vi "testItemIndexOne.vi"(8 "error in (no error)":errorcluster, 11 "TestCase in":refnum<class "ListImp_Populated.lvclass">) -> (0 "error out":errorcluster, 3 "TestCase out":refnum<class "ListImp_Populated.lvclass">)   [LabVIEW 2013, in "ListImp_Populated.lvclass"]
uses:
  ListImp_Populated.lvclass
  ListImp_Populated.lvclass/ListImp_Populated.ctl
  source/LapDog.Collections.Lists/ListImp/ListImp.lvclass
  <vilib>/addons/_JKI Toolkits/VI Tester/TestCase.llb/TestCase.lvclass
  UnitTestComparisons/UnitTestComparisons.lvlib
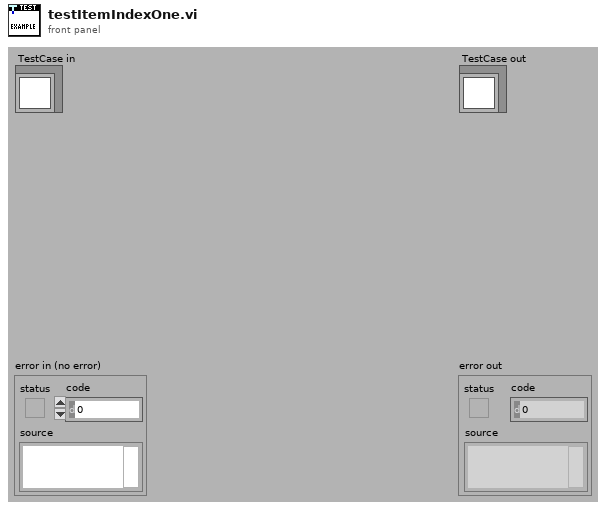
[diagram p1: front panel]
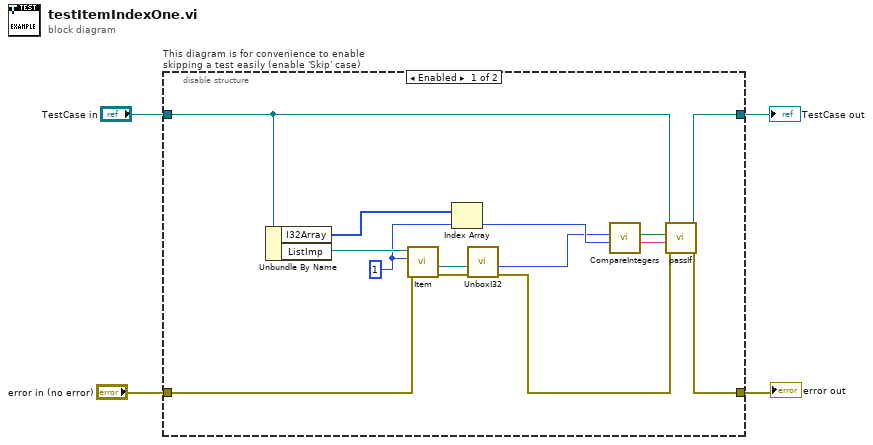
[diagram p0: block diagram]
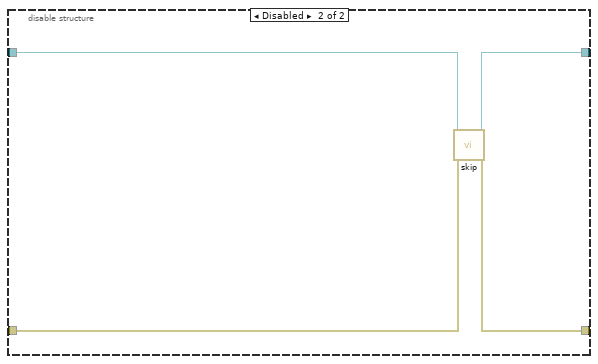
[diagram p2: hidden frame]
diagram:
  n1 = disable-structure "This diagram is for convenience to enable skipping a test easily (enable 'Skip' case)" shown="Enabled" {
    disable-tunnel: "TestCase in" -> [w13 w22]
    disable-tunnel: [w18 w20] -> w1
    disable-tunnel: [w17 w21] -> w3
    disable-tunnel: "error in (no error)" -> [w11 w19]
    frame Enabled {
      w9 = 1 ("Index")
      n2 = Unbundle By Name(w13) -> ("I32Array"=w10:i32[], "ListImp"=w14:refnum<class "ListImp.lvclass">)
      n3 = call-dynamic "Item.vi"("error in (no error)"=w11, "Index"=w9, "ListImp in"=w14) -> ("error out"=w7:errorcluster, "Item"=w8:refnum<class>)  [unwired: 6 in, 1 out]
      n4 = Index Array(array=w10, index=w9) -> (element=w12:i32)
      n5 = call "UnboxI32.vi"("error in (no error)"=w7, "Item"=w8) -> ("error out"=w6:errorcluster, "Value"=w5:i32)  [unwired: 8 in]
      n6 = call "CompareIntegers.vi"("Expected Value"=w12, "Actual Value"=w5) -> ("Message"=w15:string, "Equal?"=w16:bool)  [unwired: 8 in]
      n7 = call-dynamic "passIf.vi"("error in (no error)"=w6, "message (\"\")"=w15, "pass"=w16, "TestCase in"=w13) -> ("error out"=w17:errorcluster, "TestCase out"=w18:refnum<class "ListImp_Populated.lvclass">)  [unwired: 6 in]
    }
    frame Disabled {
      # "skip test result while test is under development"
      n8 = call <vilib>:"skip.vi"("error in (no error)"=w19, "TestCase in"=w22) -> ("error out"=w21:errorcluster, "TestCase out"=w20:refnum<class "ListImp_Populated.lvclass">)  [unwired: 8 in]
    }
  }
  "error out" <- w3
  "TestCase out" <- w1
